vi "test_libssh2_session_read_timeout.vi"() -> ()   [LabVIEW 2013, in "libssh2_integration_tests.lvlib"]
uses:
  libssh2_integration_tests.lvlib
  <vilib>/addons/_JKI Toolkits/Caraya/classes/Test/Test.lvclass
  <vilib>/addons/_JKI Toolkits/Caraya/classes/Assert/Assert.lvclass
  libssh2/libssh2.lvlib
panel:
  out "error out":errorcluster
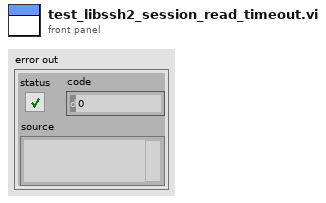
[diagram p1: front panel]
types:
  T1 = typedef "libssh2.lvlib/Session Refnum.ctl" = refnum<k1>
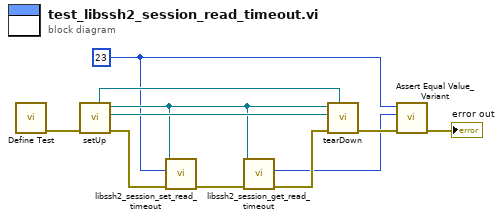
[diagram p0: block diagram]
diagram:
  w2 = 23
  n1 = call <vilib>:"Define Test.vi"() -> ("error out"=w11:errorcluster)  [unwired: 10 in, 1 out]
  n2 = call "setUp.vi"("error in (no error)"=w11) -> ("error out"=w7:errorcluster, "connection ID"=w10:refnum<k5>, "session"=w4:T1, "fixture"=w9:refnum<class "Server Fixture.lvclass">)  [unwired: 7 in]
  n3 = call "libssh2_session_set_read_timeout.vi"("error in (no error)"=w7, "read timeout in seconds (0 = default)"=w2, "session"=w4) -> ("error out"=w8:errorcluster)  [unwired: 8 in]
  n4 = call "libssh2_session_get_read_timeout.vi"("error in (no error)"=w8, "session"=w4) -> ("error out"=w5:errorcluster, "read timeout in seconds"=w3:i32)  [unwired: 8 in]
  n5 = call "tearDown.vi"("fixture"=w9, "error in (no error)"=w5, "connection ID"=w10, "session"=w4) -> ("error out"=w6:errorcluster)  [unwired: 7 in]
  n6 = call <vilib>:"Assert Equal Value_Variant.vi"("error in (no error)"=w6, "Y"=w3, "X"=w2) -> ("error out"=→"error out":errorcluster)  [unwired: 7 in, 1 out]
